vi "Set Macro Configs.vi"(8 "error in (no error)":errorcluster, 10 "Array of Macro Configs":T1[](array[typedef]), 11 "Motions Configuration in":refnum<class "Motions Configuration.lvclass">) -> (0 "error out":errorcluster, 3 "Motions Configuration out":refnum<class "Motions Configuration.lvclass">)   [LabVIEW 2016, in "Hardware.lvlib" / "Motions.lvlib" / "Motions Configuration.lvclass"]
uses:
  <userlib>/Common Components/Hardware/Abstract System/Motions/Motions Config/Motions Configuration.lvclass
  <userlib>/Common Components/Hardware/Abstract System/Motions/Motions Config/Macro Config.ctl
  <userlib>/Common Components/TriggerAction Q/TriggerAction Q/Element Data.ctl
  <userlib>/Common Components/Hardware/Abstract System/Motions/Motions Config/Motions Configuration.lvclass/Motions Configuration.ctl
  <userlib>/Common Components/Hardware/Abstract System/Motions/Motions/Motions.lvclass/Motions.ctl
  <userlib>/Common Components/TriggerAction Q/TriggerAction Q/TriggerAction Q.lvclass
  <userlib>/Common Components/Hardware/Abstract System/Motions/Motions/Motions.lvclass
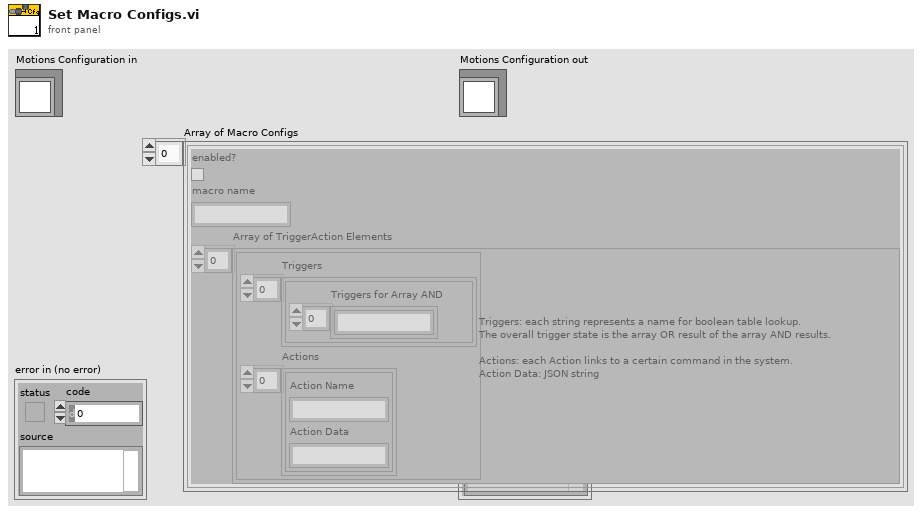
[diagram p1: front panel]
types:
  T1 = typedef "Hardware.lvlib/Motions.lvlib/Motions Configuration.lvclass/Macro Config.ctl" = cluster{"enabled?":bool, "macro name":string, "Array of TriggerAction Elements":T2[]}
  T2 = typedef "TriggerAction Q.lvclass/Element Data.ctl" = cluster{"Triggers":cluster{"Triggers for Array AND":string[]}[], "Actions":cluster{"Action Name":string, "Action Data":string}[]}
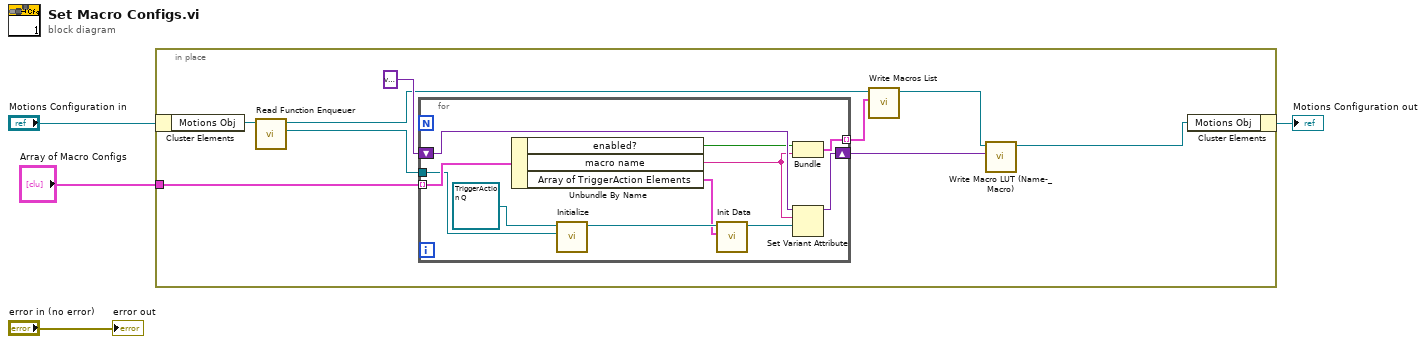
[diagram p0: block diagram]
diagram:
  n1 = in-place {
    in-place-border: "Array of Macro Configs" -> [w9]
    n2 = in-place-cluster #1("Motions Configuration in") -> ("Motions Obj"=w12:refnum<class "Motions.lvclass">)
    n3 = call <userlib>:"Read Function Enqueuer.vi"("Motions in"=w12) -> ("Actor Framework:Message Enqueuer"=w5:refnum<class "Message Enqueuer.lvclass">, "Motions out"=w6:refnum<class "Motions.lvclass">)  [unwired: 9 in]
    n4 = for {
      tunnel: w9 -> [w24] mode=indexing
      shift-right: [w18] -> w7
      shift-left: variant -> [w23]
      tunnel: [w15] -> w8 mode=indexing
      tunnel: w5 -> [w14]
      n5 = Unbundle By Name(w24) -> ("enabled?"=w17:bool, "macro name"=w16:string, "Array of TriggerAction Elements"=w20:T2[])
      n6 = call <userlib>:"Initialize.vi"("Function Enqueuer"=w14, "TriggerAction in"=refnum<class "TriggerAction Q.lvclass"> refnum ("TriggerAction Q.lvclass")) -> ("TriggerAction out"=w21:refnum<class "TriggerAction Q.lvclass">)  [unwired: 8 in, 1 out]
      n7 = call <userlib>:"Init Data.vi"("Array of TriggerAction Elements"=w20, "TriggerAction in"=w21) -> ("TriggerAction out"=w19:refnum<class "TriggerAction Q.lvclass">)  [unwired: 8 in, 1 out]
      n8 = Bundle("enabled?"=w17, "macro name"=w16) -> (w15:cluster{"enabled?":bool, "macro name":string})  [unwired: 1 in]
      n9 = Set Variant Attribute(Variant=w23, name=w16, value=w19) -> (Variant out=w18:variant)  [unwired: 1 in, 2 out]
    }
    n10 = call <userlib>:"Write Macros List.vi"("Macros List"=w8, "Motions in"=w6) -> ("Motions out"=w13:refnum<class "Motions.lvclass">)  [unwired: 9 in]
    n11 = call <userlib>:"Write Macro LUT (Name-_Macro).vi"("Macro LUT (Name->Macro)"=w7, "Motions in"=w13) -> ("Motions out"=w11:refnum<class "Motions.lvclass">)  [unwired: 9 in]
    n12 = in-place-cluster #1("Motions Obj"=w11) -> (→"Motions Configuration out":refnum<class "Motions Configuration.lvclass">)
  }
  "error out" <- "error in (no error)"
